vi "DAQ-Abort FGV.vi"(7 "Finished":bool, 11 "error in (no error)":errorcluster, 13 "Action":enum16{"Default", "Init", "Abort", "1st error"}(ring)) -> (8 "Stop":bool, 10 "Was aborted":bool, 15 "Errors":errorcluster)   [LabVIEW 2020]
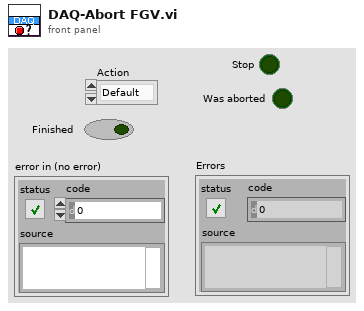
[diagram p1: front panel]
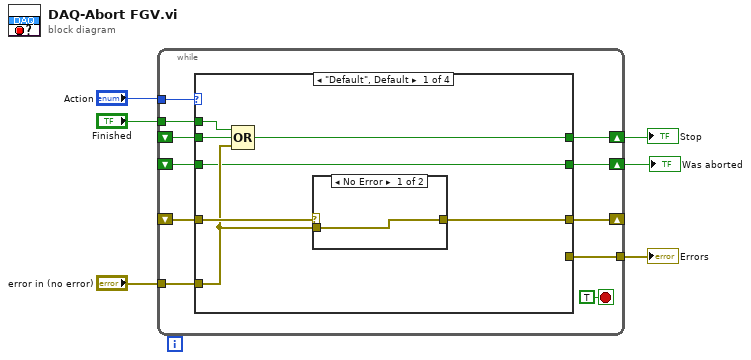
[diagram p0: block diagram]
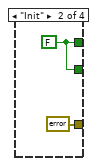
[diagram p3: hidden frame]
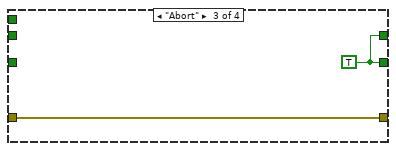
[diagram p4: hidden frame]
diagram:
  n1 = while {
    tunnel: "Action" -> [w17]
    shift-right: [w16] -> w6
    shift-left: _ -> [w15]
    tunnel: "Finished" -> [w14]
    tunnel: "error in (no error)" -> [w13]
    shift-right: [w12] -> _
    shift-left: _ -> [w11]
    tunnel: [w9] -> w3
    shift-right: [w8] -> w1
    shift-left: _ -> [w7]
    stop <- TRUE stop-if-true
    n2 = case shown="\"Default\", Default" w17 {
      tunnel: [w24 w27 w29 w31] -> w16
      tunnel: w15 -> [w23 _ _ w31]
      tunnel: w14 -> [w22 _ _ _]
      tunnel: w13 -> [w19 _ _ _]
      tunnel: [w20 errorcluster {"status"=FALSE, "code"=0, "source"=""} ("error constant") w30 w33] -> w12
      tunnel: w11 -> [w21 _ w30 w33]
      tunnel: [_ _ _ w33] -> w9
      tunnel: [w18 w27 w29 w32] -> w8
      tunnel: w7 -> [w18 _ _ w32]
      frame "Default", Default {
        n3 = Compound Arithmetic op=OR(w22, w23, w19) -> (w24:bool)
        n4 = case shown="No Error" w21 {
          selector: w21 -> [_ w26]
          tunnel: [w25 w26] -> w20
          tunnel: w19 -> [w25 _]
          frame No Error {
          }
          frame Error {
          }
        }
      }
      frame "Init" {
        w27 = FALSE
      }
      frame "Abort" {
        w29 = TRUE
      }
      frame "1st error" {
      }
    }
  }
  "Stop" <- w6
  "Errors" <- w3
  "Was aborted" <- w1
